vi "Ramp Time Completions.vi"(2 "Current Ramp Time":u64, 3 "Initial":T1) -> (0 "Still in Ramp":bool, 1 "Fraction\nCompleted":dbl)   [LabVIEW 2009]
uses:
  Ramp Time Tuple.ctl
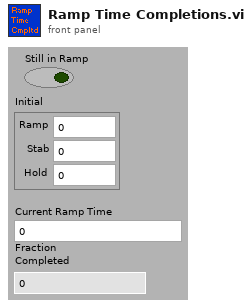
[diagram p1: front panel]
types:
  T1 = typedef "Ramp Time Tuple.ctl" = cluster{"Ramp":dbl, "Stab":dbl, "Hold":dbl}
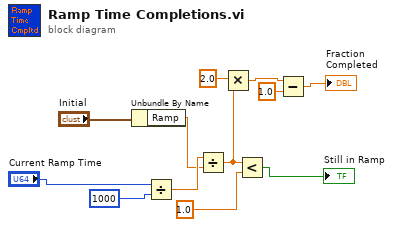
[diagram p0: block diagram]
diagram:
  n1 = Unbundle By Name("Initial") -> ("Ramp"=w9:dbl)
  n2 = Divide(x="Current Ramp Time", y=u32 1000) -> (x/y=w10:dbl)
  n3 = Divide(x=w10, y=w9) -> (x/y=w2:dbl)
  n4 = Multiply(x=2.0, y=w2) -> (x*y=w5:dbl)
  n5 = Less?(x=w2, y=1.0) -> (x < y?=→"Still in Ramp":bool)
  n6 = Subtract(x=w5, y=1.0) -> (x-y=→"Fraction\nCompleted":dbl)
